vi "AIT 664 - Extract Tx Ports from System Explorer.vi"(0 "Found Output VL":T2, 5 "Item Refs":T1[](array[typedef]) format="%.0x", 7 "VL Id Found?":bool, 9 "Output VLs":T2[](array[typedef]), 11 "error in (no error)":errorcluster) -> (4 "Output VLs out":T2[](array[typedef]), 15 "error out":errorcluster)   [LabVIEW 2013, in "AIT 664 Custom Device.lvlib"]
doc: "Extraxt the Tx ports from the system explorer and return the parameters defined by the user"
uses:
  AIT 664 Custom Device.lvlib
  Controls/664 - XML Output VL.ctl
  Controls/664 - XML Tx Message Port.ctl
  Controls/664 - Sampling Type.ctl
  Controls/664 -Param.ctl
  <vilib>/NI Veristand/Custom Device API/Custom Device Item Ref.ctl
  Controls and Global/Global.vi
  <vilib>/NI Veristand/Custom Device API/Get Item Property (U32).vi
  <vilib>/NI Veristand/Custom Device API/Custom Device API.lvlib
  <vilib>/NI Veristand/Custom Device Tools/Custom Device Utility Library/Custom Device Utility Library.lvlib
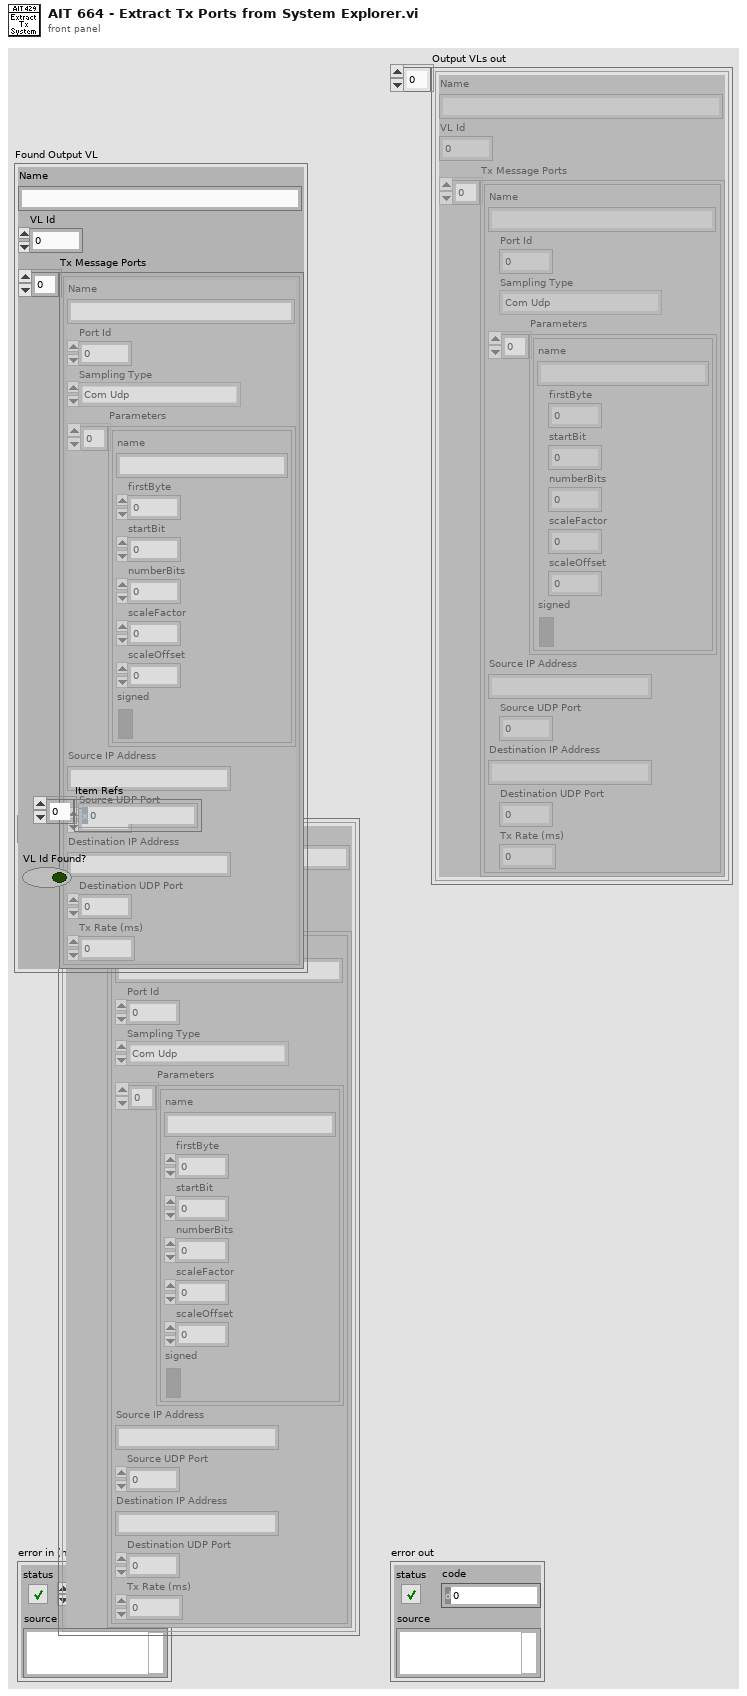
[diagram p1: front panel]
types:
  T1 = typedef "Custom Device API.lvlib/Custom Device Item Ref.ctl" = u64
  T2 = typedef "AIT 664 Custom Device.lvlib/664 - XML Output VL.ctl" = cluster{"Name":string, "VL Id":u32, "Tx Message Ports":T3[]}
  T3 = typedef "AIT 664 Custom Device.lvlib/664 - XML Tx Message Port.ctl" = cluster{"Name":string, "Port Id":u32, "Sampling Type":T4, "Parameters":T5[], "Source IP Address":string, "Source UDP Port":u32, "Destination IP Address":string, "Destination UDP Port":u32, "Tx Rate (ms)":u32}
  T4 = typedef "AIT 664 Custom Device.lvlib/664 - Sampling Type.ctl" = enum16{"Com Udp", "Com Udp Queuing", "Sap Udp", "Sap Ip", "Sap Mac", "Unknown"}
  T5 = typedef "AIT 664 Custom Device.lvlib/664 -Param.ctl" = cluster{"name":string, "firstByte":i32, "startBit":i32, "numberBits":i32, "scaleFactor":dbl, "scaleOffset":dbl, "signed":bool}
  T6 = typedef "Custom Device API.lvlib/Custom Device Item Info.ctl" = cluster{"Name":string, "Is Channel":bool, "GUID":string, "Is Waveform":bool}
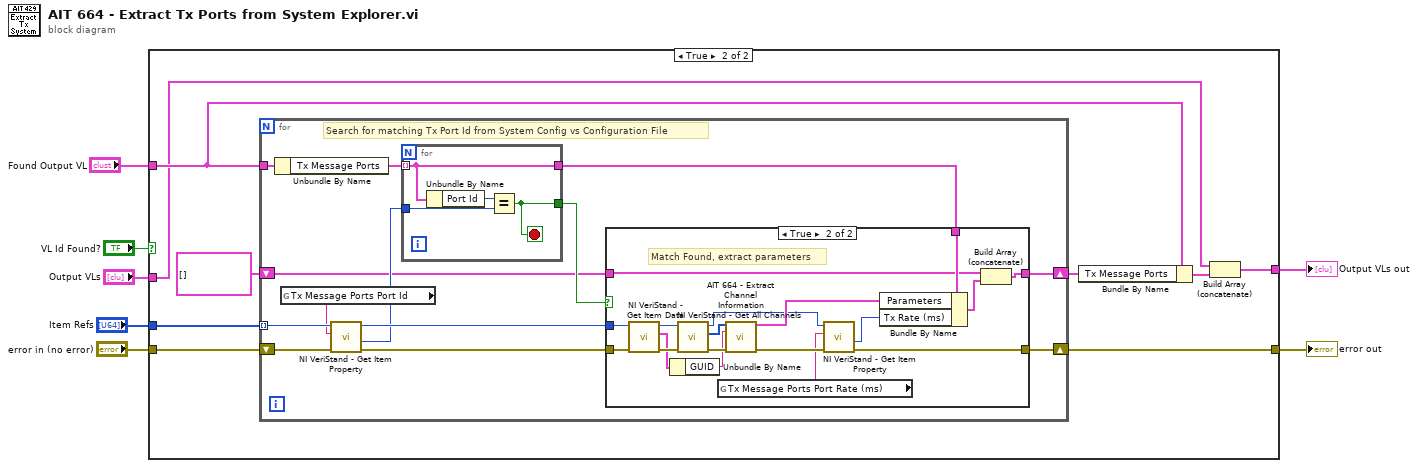
[diagram p0: block diagram]
diagram:
  n1 = case shown="True" "VL Id Found?" {
    tunnel: "Item Refs" -> [_ w18]
    tunnel: "Found Output VL" -> [_ w16]
    tunnel: "Output VLs" -> [w9 w14]
    tunnel: [w9 w12] -> w5
    tunnel: "error in (no error)" -> [w8 w11]
    tunnel: [w8 w10] -> w7
    frame False {
    }
    frame True {
      n2 = for {
        tunnel: w18 -> [w31] mode=indexing
        tunnel: w16 -> [w27]
        shift-right: [w21] -> w15
        shift-left: T3[] [] -> [w22]
        shift-right: [w20] -> w10
        shift-left: w11 -> [w19]
        # "Search for matching Tx Port Id from System Config vs Configuration File"
        n3 = Unbundle By Name(w27) -> ("Tx Message Ports"=w26:T3[])
        n4 = global read "Global.vi" "Tx Message Ports Port Id"() -> (w30:string)
        n5 = call-poly <vilib>:"NI VeriStand - Get Item Property.vi"("error in (no error)"=w19, "Property Name"=w30, "Item Ref in"=w31) -> ("error out"=w29:errorcluster, "Value"=w25:u32, "Item Ref out"=w28:T1)  [unwired: 5 in, 1 out]
        n6 = for {
          tunnel: w26 -> [w52] mode=indexing
          tunnel: w25 -> [w54]
          tunnel: [w53] -> w24
          tunnel: [w52] -> w23
          stop <- w53 stop-if-true
          n7 = Unbundle By Name(w52) -> ("Port Id"=w55:u32)
          n8 = Equal?(x=w55, y=w54) -> (x = y?=w53:bool)
        }
        n9 = case shown="True" w24 {
          tunnel: w29 -> [w32 w44]
          tunnel: w28 -> [_ w42]
          tunnel: w23 -> [_ w49]
          tunnel: w22 -> [w33 w47]
          tunnel: [w33 w45] -> w21
          tunnel: [w32 w37] -> w20
          frame False {
          }
          frame True {
            # "Match Found, extract parameters"
            n10 = call <vilib>:"NI VeriStand - Get Item Data.vi"("error in (no error)"=w44, "Item Ref in"=w42) -> ("error out"=w43:errorcluster, "Item Info"=w40:T6, "Item Ref out"=w41:T1)  [unwired: 6 in, 1 out]
            n11 = Unbundle By Name(w40) -> ("GUID"=w39:string)
            n12 = call <vilib>:"NI VeriStand - Get All Channels.vi"("error in"=w43, "Section Ref in"=w41) -> ("error out"=w50:errorcluster, "Channel Refs"=w51:T1[], "Section Ref out"=w35:T1)  [unwired: 6 in, 1 out]
            n13 = global read "Global.vi" "Tx Message Ports Port Rate (ms)"() -> (w34:string)
            n14 = call "AIT 664 - Extract Channel Information.vi"("Channel Refs"=w51, "Parent Guid"=w39, "error in (no error)"=w50) -> ("Parameters out"=w48:T5[], "error out"=w38:errorcluster)  [unwired: 11 in]
            n15 = call-poly <vilib>:"NI VeriStand - Get Item Property.vi"("error in (no error)"=w38, "Property Name"=w34, "Item Ref in"=w35) -> ("error out"=w37:errorcluster, "Value"=w36:u32)  [unwired: 5 in, 2 out]
            n16 = Bundle By Name(cluster=w49, "Parameters"=w48, "Tx Rate (ms)"=w36) -> (w46:T3)
            n17 = Build Array (concatenate)(w47, w46) -> (w45:T3[])
          }
        }
      }
      n18 = Bundle By Name(cluster=w16, "Tx Message Ports"=w15) -> (w13:T2)
      n19 = Build Array (concatenate)(w14, w13) -> (w12:T2[])
    }
  }
  "error out" <- w7
  "Output VLs out" <- w5
